vi "Core_2018-02-21.vi"(5 "Error In":errorcluster) -> (19 "Error Out":errorcluster)   [LabVIEW 2017]
uses:
  <vilib>/Platform/TimedLoop/XDataNode/timing_clust.ctl
  <vilib>/Platform/TimedLoop/XDataNode/nitl_modes.ctl
  <vilib>/Platform/TimedLoop/XDataNode/wakeup.ctl
  <vilib>/Platform/TimedLoop/XDataNode/XDataNode.xnode
  <vilib>/Platform/TimedLoop/XDataNode/XDNodeRunTimeDep.lvlib
panel:
  out "Heater Resistance":dbl
  # "Core Module DIagnostics"
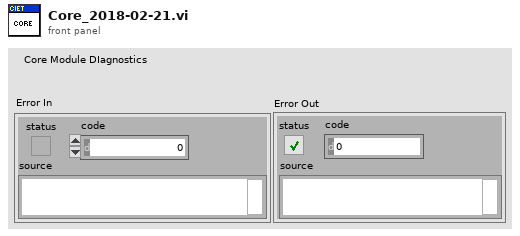
[diagram p1: front panel]
types:
  T1 = typedef "XDNodeRunTimeDep.lvlib/timing_clust.ctl" = cluster{"Expected End [f-1]":u64, "Actual End [f-1]":u64, "Finished Late? [f-1]":bool, "Expected End [i-1]":u64, "Actual End [i-1]":u64, "Finished Late? [i-1]":bool, "Expected Start [i]":u64, "Actual Start [i]":u64, "Expected Start [f]":u64, "Actual Start [f]":u64, "Source Name":string, "Structure Name":string, "Period":i64, "Deadline":i64, "Offset":i64, "Start":i64, "Priority":i32, "Timeout":i32, "Mode":T2, "Wakeup Reason":T3, "Error":errorcluster, "Source Type":string, "Secondary Source Type":string, "Global End Time":u64, "Global Start Time":u64, "Frame Duration":u64, "Iteration Duration":u64, "Assigned CPU":i32, "I/O Scan Engine Mode":u32}
  T2 = typedef "XDNodeRunTimeDep.lvlib/nitl_modes.ctl" = enum32{"No Change", "Process missed periods, maintain original phase", "Discard missed periods, maintain original phase", "Process missed periods, ignore original phase", "Discard missed periods, ignore original phase"}
  T3 = typedef "XDNodeRunTimeDep.lvlib/wakeup.ctl" = enum32{"Normal", "Aborted", "Asynchronous wakeup", "Timing source error", "Timed loop error", "Timeout"}
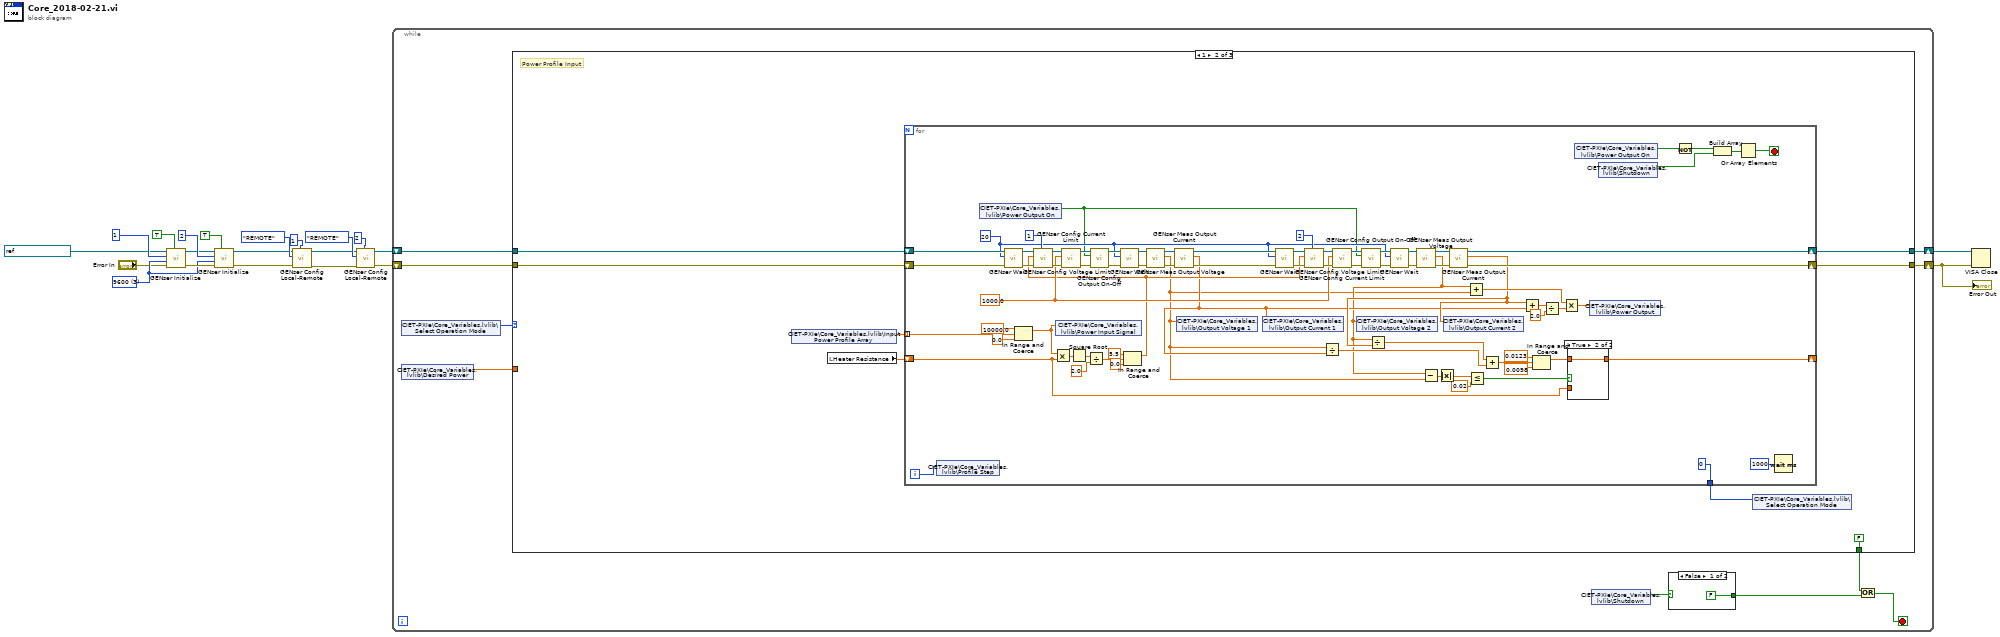
[diagram p0: block diagram]
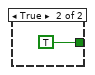
[diagram p2: hidden frame]
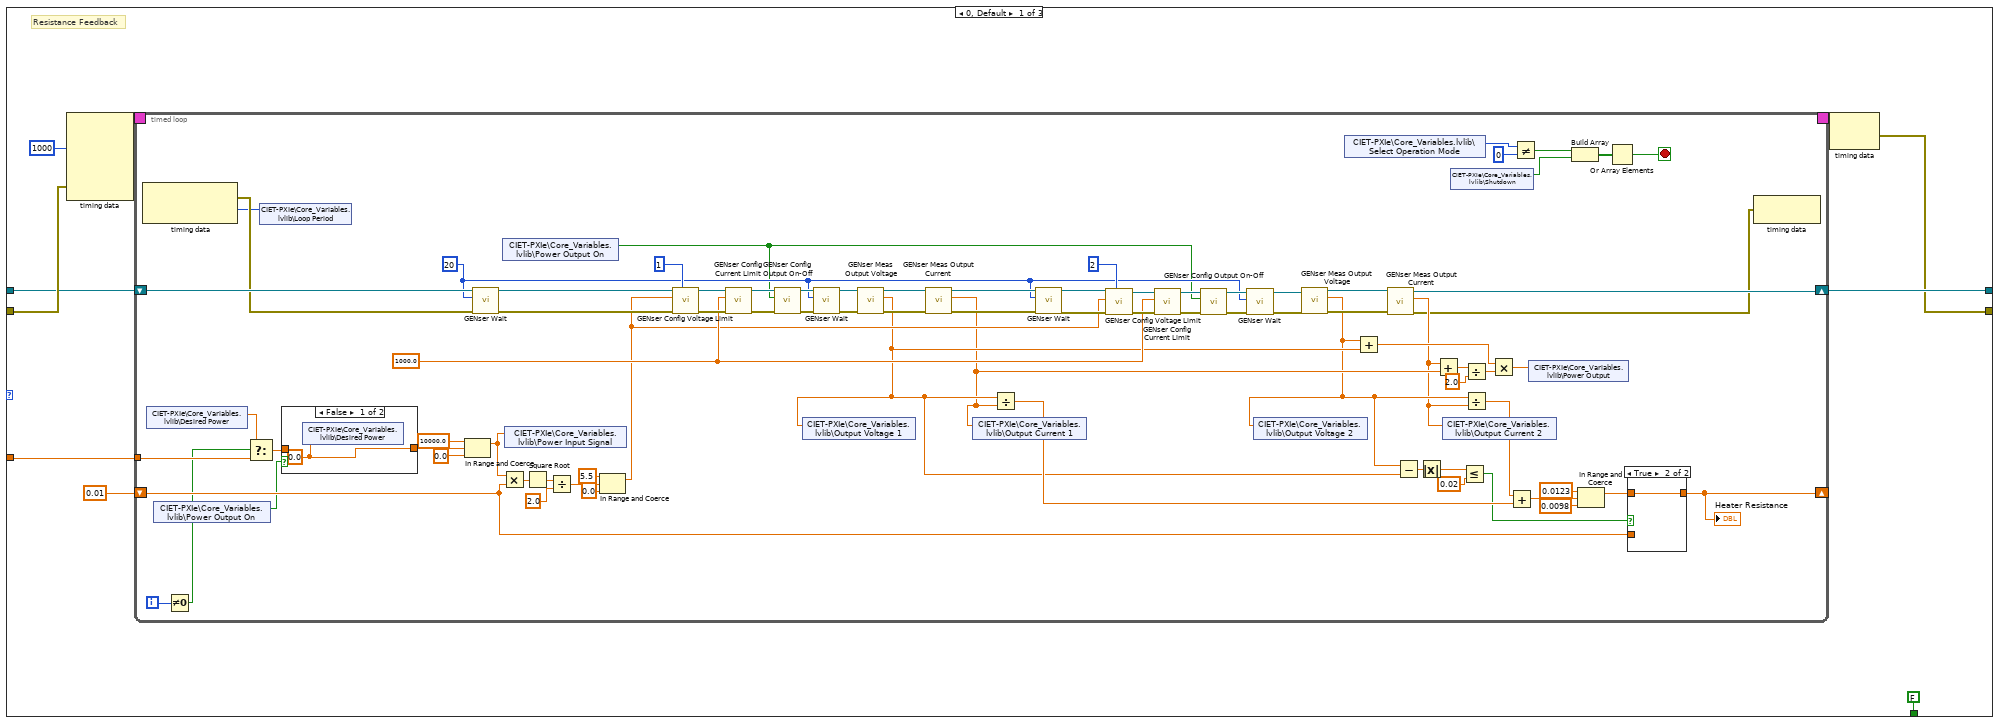
[diagram p3: hidden frame]
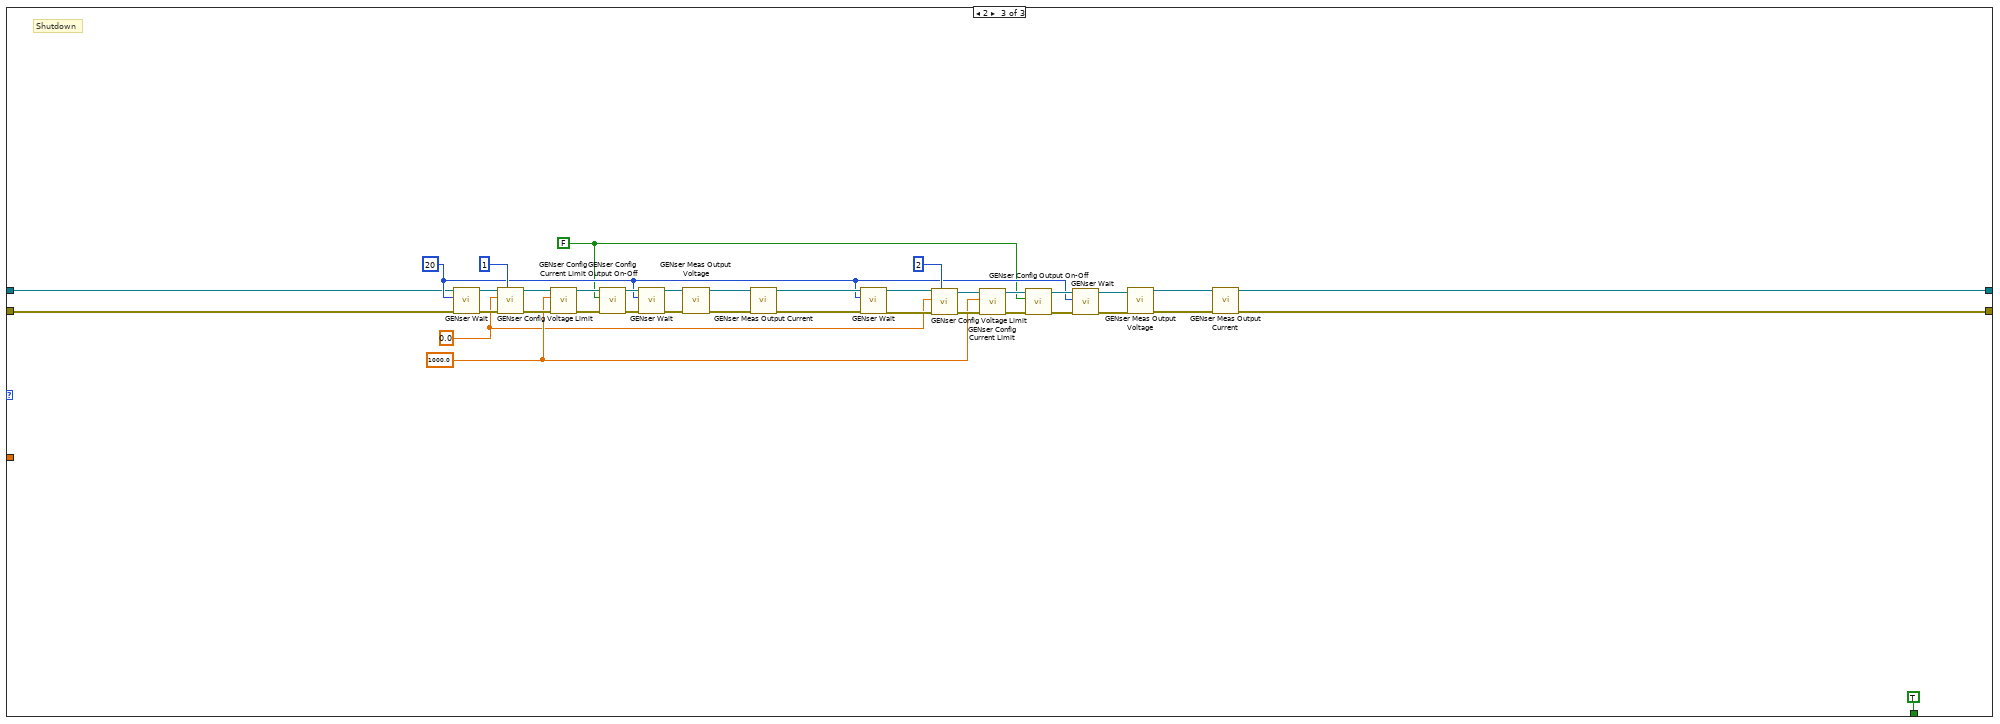
[diagram p7: hidden frame]
diagram:
  w7 = u16 3 items=["1200", "2400", "4800", "9600", "19200"] ("BAUD")
  n1 = call "GENser Initialize.vi"("Reset (T)"=TRUE, "error in (no error)"="Error In", "BAUD"=w7, "GEN Addr"=i16 1, "VISA name"=refnum<visa-resource-name> "Power_Supplies") -> ("error out"=w16:errorcluster, "VISA out"=w17:refnum<visa-resource-name>)  [unwired: 5 in]
  n2 = call "GENser Initialize.vi"("Reset (T)"=TRUE, "error in (no error)"=w16, "BAUD"=w7, "GEN Addr"=i16 2, "VISA name"=w17) -> ("error out"=w13:errorcluster, "VISA out"=w14:refnum<visa-resource-name>)  [unwired: 5 in]
  n3 = call "GENser Config Local-Remote.vi"("GEN Addr"=i16 1, "error"=w13, "Mode"=enum16{"LOCAL", "REMOTE", "LOCKOUT"}."REMOTE", "VISA"=w14) -> ("error out"=w8:errorcluster, "VISA out"=w9:refnum<visa-resource-name>)  [unwired: 6 in]
  n4 = call "GENser Config Local-Remote.vi"("GEN Addr"=i16 2, "error"=w8, "Mode"=enum16{"LOCAL", "REMOTE", "LOCKOUT"}."REMOTE", "VISA"=w9) -> ("error out"=w5:errorcluster, "VISA out"=w4:refnum<visa-resource-name>)  [unwired: 6 in]
  n5 = while {
    shift-right: [w28] -> w1
    shift-left: w5 -> [w31]
    shift-right: [w29] -> w2
    shift-left: w4 -> [w30]
    stop <- w22 stop-if-true
    n6 = shared-variable "CIET-PXIe\\Core_Variables.lvlib\\Select Operation Mode"() -> (w27:i32)  [unwired: 1 in, 1 out]
    n7 = shared-variable "CIET-PXIe\\Core_Variables.lvlib\\Desired Power"() -> (w26:dbl)  [unwired: 1 in, 1 out]
    n8 = case shown="1" w27 {
      tunnel: w31 -> [w41 w144 w228]
      tunnel: w30 -> [w40 w147 w227]
      tunnel: [w38 w146 w226] -> w29
      tunnel: [w37 w143 w225] -> w28
      tunnel: [FALSE ("Shutdown") FALSE ("Shutdown") TRUE ("Shutdown")] -> w24
      tunnel: w26 -> [w35 _ _]
      frame 0, Default {
        # "Resistance Feedback"
        n9 = node-c288(i64 1000 ("Period"), w41) -> (w43:T1)  [unwired: 3 in]
        n10 = timed-loop {
          timing: w43 -> [_]
          timing-out: [_] -> w42
          shift-right: [w45] -> w38
          shift-left: w40 -> [w110]
          shift-right: [w66] -> _
          shift-left: 0.01 -> [w77]
          tunnel: w35 -> [w62]
          i -> [w64]
          stop <- w58 stop-if-true
          w82 = u32 20 ("Delay (20 mS)")
          w95 = 1000.0 ("Current Limit")
          n11 = node-c288() -> (w109:errorcluster, w56:i64)  [unwired: 1 in]
          n12 = shared-variable "CIET-PXIe\\Core_Variables.lvlib\\Desired Power"() -> (w57:dbl)  [unwired: 1 in, 1 out]
          n13 = shared-variable "CIET-PXIe\\Core_Variables.lvlib\\Power Output On"() -> (w54:bool)  [unwired: 1 in, 1 out]
          n14 = Not Equal To 0?(x=w64) -> (x != 0?=w61:bool)
          n15 = Select(t=w57, s=w61, f=w62) -> (s? t:f=w63:dbl)
          n16 = shared-variable "CIET-PXIe\\Core_Variables.lvlib\\Loop Period"(w56) -> ()  [unwired: 1 in, 1 out]
          n17 = case shown="False" w54 {
            tunnel: [w124 w125] -> w86
            tunnel: w63 -> [_ w125]
            frame False {
              w124 = 0.0 ("Desired Power")
              n18 = shared-variable "CIET-PXIe\\Core_Variables.lvlib\\Desired Power"(w124) -> ()  [unwired: 1 in, 1 out]
            }
            frame True {
            }
          }
          n19 = In Range and Coerce(upper limit=10000.0, x=w86, lower limit=0.0) -> (coerced(x)=w53:dbl)  [unwired: 1 out]
          n20 = call "GENser Wait.vi"("error"=w109, "Delay (20 mS)"=w82, "VISA"=w110) -> ("error out"=w111:errorcluster, "VISA out"=w108:refnum<visa-resource-name>)  [unwired: 7 in]
          n21 = Multiply(x=w53, y=w77) -> (x*y=w92:dbl)
          n22 = shared-variable "CIET-PXIe\\Core_Variables.lvlib\\Power Output On"() -> (w55:bool)  [unwired: 1 in, 1 out]
          n23 = shared-variable "CIET-PXIe\\Core_Variables.lvlib\\Power Input Signal"(w53) -> ()  [unwired: 1 in, 1 out]
          n24 = Square Root(x=w92) -> (sqrt(x)=w91:dbl)
          n25 = Divide(x=w91, y=2.0) -> (x/y=w87:dbl)
          n26 = In Range and Coerce(upper limit=5.5, x=w87, lower limit=0.0) -> (coerced(x)=w85:dbl)  [unwired: 1 out]
          n27 = call "GENser Config Voltage Limit.vi"("GEN Addr"=i16 1, "error"=w111, "Volt Limit"=w85, "VISA"=w108) -> ("error out"=w123:errorcluster, "VISA out"=w107:refnum<visa-resource-name>)  [unwired: 6 in]
          n28 = call "GENser Config Current Limit.vi"("error"=w123, "Current Limit"=w95, "VISA"=w107) -> ("error out"=w120:errorcluster, "VISA out"=w106:refnum<visa-resource-name>)  [unwired: 7 in]
          n29 = call "GENser Config Output On-Off.vi"("error"=w120, "Output ON"=w55, "VISA"=w106) -> ("error out"=w118:errorcluster, "VISA out"=w105:refnum<visa-resource-name>)  [unwired: 7 in]
          n30 = call "GENser Wait.vi"("error"=w118, "Delay (20 mS)"=w82, "VISA"=w105) -> ("error out"=w117:errorcluster, "VISA out"=w104:refnum<visa-resource-name>)  [unwired: 7 in]
          n31 = call "GENser Meas Output Voltage.vi"("error"=w117, "VISA"=w104) -> ("error out"=w119:errorcluster, "Output Voltage"=w50:dbl, "VISA out"=w103:refnum<visa-resource-name>)  [unwired: 7 in]
          n32 = shared-variable "CIET-PXIe\\Core_Variables.lvlib\\Output Voltage 1"(w50) -> ()  [unwired: 1 in, 1 out]
          n33 = call "GENser Meas Output Current.vi"("error"=w119, "VISA"=w103) -> ("error out"=w115:errorcluster, "Output Current"=w49:dbl, "VISA out"=w102:refnum<visa-resource-name>)  [unwired: 7 in]
          n34 = shared-variable "CIET-PXIe\\Core_Variables.lvlib\\Output Current 1"(w49) -> ()  [unwired: 1 in, 1 out]
          n35 = Divide(x=w50, y=w49) -> (x/y=w69:dbl)
          n36 = call "GENser Wait.vi"("error"=w115, "Delay (20 mS)"=w82, "VISA"=w102) -> ("error out"=w114:errorcluster, "VISA out"=w101:refnum<visa-resource-name>)  [unwired: 7 in]
          n37 = call "GENser Config Voltage Limit.vi"("GEN Addr"=i16 2, "error"=w114, "Volt Limit"=w85, "VISA"=w101) -> ("error out"=w116:errorcluster, "VISA out"=w100:refnum<visa-resource-name>)  [unwired: 6 in]
          n38 = call "GENser Config Current Limit.vi"("error"=w116, "Current Limit"=w95, "VISA"=w100) -> ("error out"=w113:errorcluster, "VISA out"=w99:refnum<visa-resource-name>)  [unwired: 7 in]
          n39 = call "GENser Config Output On-Off.vi"("error"=w113, "Output ON"=w55, "VISA"=w99) -> ("error out"=w122:errorcluster, "VISA out"=w98:refnum<visa-resource-name>)  [unwired: 7 in]
          n40 = call "GENser Wait.vi"("error"=w122, "Delay (20 mS)"=w82, "VISA"=w98) -> ("error out"=w112:errorcluster, "VISA out"=w97:refnum<visa-resource-name>)  [unwired: 7 in]
          n41 = call "GENser Meas Output Voltage.vi"("error"=w112, "VISA"=w97) -> ("error out"=w121:errorcluster, "Output Voltage"=w48:dbl, "VISA out"=w96:refnum<visa-resource-name>)  [unwired: 7 in]
          n42 = shared-variable "CIET-PXIe\\Core_Variables.lvlib\\Output Voltage 2"(w48) -> ()  [unwired: 1 in, 1 out]
          n43 = shared-variable "CIET-PXIe\\Core_Variables.lvlib\\Select Operation Mode"() -> (w52:i32)  [unwired: 1 in, 1 out]
          n44 = Add(x=w48, y=w50) -> (x+y=w78:dbl)
          n45 = call "GENser Meas Output Current.vi"("error"=w121, "VISA"=w96) -> ("error out"=w44:errorcluster, "Output Current"=w47:dbl, "VISA out"=w45:refnum<visa-resource-name>)  [unwired: 7 in]
          n46 = Subtract(x=w48, y=w50) -> (x-y=w73:dbl)
          n47 = Absolute Value(x=w73) -> (abs(x)=w72:dbl)
          n48 = Add(x=w47, y=w49) -> (x+y=w81:dbl)
          n49 = shared-variable "CIET-PXIe\\Core_Variables.lvlib\\Output Current 2"(w47) -> ()  [unwired: 1 in, 1 out]
          n50 = shared-variable "CIET-PXIe\\Core_Variables.lvlib\\Shutdown"() -> (w51:bool)  [unwired: 1 in, 1 out]
          n51 = Less Or Equal?(x=w72, y=0.02) -> (x <= y?=w68:bool)
          n52 = Divide(x=w81, y=2.0) -> (x/y=w79:dbl)
          n53 = Divide(x=w48, y=w47) -> (x/y=w70:dbl)
          n54 = Multiply(x=w78, y=w79) -> (x*y=w46:dbl)
          n55 = Add(x=w70, y=w69) -> (x+y=w74:dbl)
          n56 = Not Equal?(x=w52, y=u16 0) -> (x != y?=w60:bool)
          n57 = shared-variable "CIET-PXIe\\Core_Variables.lvlib\\Power Output"(w46) -> ()  [unwired: 1 in, 1 out]
          n58 = Build Array(w60, w51) -> (w59:bool[])
          n59 = In Range and Coerce(upper limit=0.0123, x=w74, lower limit=0.0098) -> (coerced(x)=w67:dbl)  [unwired: 1 out]
          n60 = Or Array Elements(Boolean array=w59) -> (logical OR=w58:bool)
          n61 = case shown="True" w68 {
            tunnel: w67 -> [_ w133]
            tunnel: [w132 w133] -> w66
            tunnel: w77 -> [w132 _]
            frame False {
            }
            frame True {
            }
          }
          "Heater Resistance" <- w66
          n62 = node-c288(w44) -> ()  [unwired: 1 out]
        }
        n63 = node-c288(w42) -> (w37:errorcluster)
      }
      frame 1 {
        # "Power Profile Input"
        n64 = shared-variable "CIET-PXIe\\Core_Variables.lvlib\\Input Power Profile Array"() -> (w140:dbl[])  [unwired: 1 in, 1 out]
        n65 = local read "Heater Resistance"() -> (w145:dbl)
        n66 = for {
          shift-right: [w169] -> w146
          shift-left: w147 -> [w209]
          shift-right: [w168] -> w143
          shift-left: w144 -> [w177]
          tunnel: w140 -> [w174] mode=indexing
          tunnel: [u16 0 ("y")] -> w141
          shift-right: [w149] -> _
          shift-left: w145 -> [w148]
          i -> [w164]
          stop <- w175 stop-if-true
          w184 = u32 20 ("Delay (20 mS)")
          w195 = 1000.0 ("Current Limit")
          n67 = shared-variable "CIET-PXIe\\Core_Variables.lvlib\\Profile Step"(w164) -> ()  [unwired: 1 in, 1 out]
          n68 = shared-variable "CIET-PXIe\\Core_Variables.lvlib\\Power Output On"() -> (w171:bool)  [unwired: 1 in, 1 out]
          n69 = call "GENser Wait.vi"("error"=w177, "Delay (20 mS)"=w184, "VISA"=w209) -> ("error out"=w210:errorcluster, "VISA out"=w208:refnum<visa-resource-name>)  [unwired: 7 in]
          n70 = In Range and Coerce(upper limit=10000.0, x=w174, lower limit=0.0) -> (coerced(x)=w172:dbl)  [unwired: 1 out]
          n71 = Multiply(x=w172, y=w148) -> (x*y=w192:dbl)
          n72 = shared-variable "CIET-PXIe\\Core_Variables.lvlib\\Power Input Signal"(w172) -> ()  [unwired: 1 in, 1 out]
          n73 = Square Root(x=w192) -> (sqrt(x)=w191:dbl)
          n74 = Divide(x=w191, y=2.0) -> (x/y=w187:dbl)
          n75 = In Range and Coerce(upper limit=5.5, x=w187, lower limit=0.0) -> (coerced(x)=w179:dbl)  [unwired: 1 out]
          n76 = call "GENser Config Voltage Limit.vi"("GEN Addr"=i16 1, "error"=w210, "Volt Limit"=w179, "VISA"=w208) -> ("error out"=w222:errorcluster, "VISA out"=w207:refnum<visa-resource-name>)  [unwired: 6 in]
          n77 = call "GENser Config Current Limit.vi"("error"=w222, "Current Limit"=w195, "VISA"=w207) -> ("error out"=w219:errorcluster, "VISA out"=w206:refnum<visa-resource-name>)  [unwired: 7 in]
          n78 = call "GENser Config Output On-Off.vi"("error"=w219, "Output ON"=w171, "VISA"=w206) -> ("error out"=w217:errorcluster, "VISA out"=w205:refnum<visa-resource-name>)  [unwired: 7 in]
          n79 = call "GENser Wait.vi"("error"=w217, "Delay (20 mS)"=w184, "VISA"=w205) -> ("error out"=w216:errorcluster, "VISA out"=w204:refnum<visa-resource-name>)  [unwired: 7 in]
          n80 = call "GENser Meas Output Voltage.vi"("error"=w216, "VISA"=w204) -> ("error out"=w218:errorcluster, "Output Voltage"=w150:dbl, "VISA out"=w203:refnum<visa-resource-name>)  [unwired: 7 in]
          n81 = call "GENser Meas Output Current.vi"("error"=w218, "VISA"=w203) -> ("error out"=w214:errorcluster, "Output Current"=w154:dbl, "VISA out"=w202:refnum<visa-resource-name>)  [unwired: 7 in]
          n82 = shared-variable "CIET-PXIe\\Core_Variables.lvlib\\Output Voltage 1"(w150) -> ()  [unwired: 1 in, 1 out]
          n83 = shared-variable "CIET-PXIe\\Core_Variables.lvlib\\Output Current 1"(w154) -> ()  [unwired: 1 in, 1 out]
          n84 = call "GENser Wait.vi"("error"=w214, "Delay (20 mS)"=w184, "VISA"=w202) -> ("error out"=w213:errorcluster, "VISA out"=w201:refnum<visa-resource-name>)  [unwired: 7 in]
          n85 = call "GENser Config Voltage Limit.vi"("GEN Addr"=i16 2, "error"=w213, "Volt Limit"=w179, "VISA"=w201) -> ("error out"=w215:errorcluster, "VISA out"=w200:refnum<visa-resource-name>)  [unwired: 6 in]
          n86 = Divide(x=w150, y=w154) -> (x/y=w152:dbl)
          n87 = call "GENser Config Current Limit.vi"("error"=w215, "Current Limit"=w195, "VISA"=w200) -> ("error out"=w212:errorcluster, "VISA out"=w199:refnum<visa-resource-name>)  [unwired: 7 in]
          n88 = call "GENser Config Output On-Off.vi"("error"=w212, "Output ON"=w171, "VISA"=w199) -> ("error out"=w221:errorcluster, "VISA out"=w198:refnum<visa-resource-name>)  [unwired: 7 in]
          n89 = call "GENser Wait.vi"("error"=w221, "Delay (20 mS)"=w184, "VISA"=w198) -> ("error out"=w211:errorcluster, "VISA out"=w197:refnum<visa-resource-name>)  [unwired: 7 in]
          n90 = call "GENser Meas Output Voltage.vi"("error"=w211, "VISA"=w197) -> ("error out"=w220:errorcluster, "Output Voltage"=w151:dbl, "VISA out"=w196:refnum<visa-resource-name>)  [unwired: 7 in]
          n91 = shared-variable "CIET-PXIe\\Core_Variables.lvlib\\Output Voltage 2"(w151) -> ()  [unwired: 1 in, 1 out]
          n92 = Subtract(x=w151, y=w150) -> (x-y=w160:dbl)
          n93 = Absolute Value(x=w160) -> (abs(x)=w159:dbl)
          n94 = call "GENser Meas Output Current.vi"("error"=w220, "VISA"=w196) -> ("error out"=w168:errorcluster, "Output Current"=w155:dbl, "VISA out"=w169:refnum<visa-resource-name>)  [unwired: 7 in]
          n95 = Divide(x=w151, y=w155) -> (x/y=w153:dbl)
          n96 = shared-variable "CIET-PXIe\\Core_Variables.lvlib\\Output Current 2"(w155) -> ()  [unwired: 1 in, 1 out]
          n97 = Add(x=w151, y=w150) -> (x+y=w180:dbl)
          n98 = Less Or Equal?(x=w159, y=0.02) -> (x <= y?=w157:bool)
          n99 = Add(x=w153, y=w152) -> (x+y=w161:dbl)
          n100 = Add(x=w155, y=w154) -> (x+y=w183:dbl)
          n101 = In Range and Coerce(upper limit=0.0123, x=w161, lower limit=0.0098) -> (coerced(x)=w156:dbl)  [unwired: 1 out]
          n102 = Divide(x=w183, y=2.0) -> (x/y=w181:dbl)
          n103 = Multiply(x=w180, y=w181) -> (x*y=w170:dbl)
          n104 = case shown="True" w157 {
            tunnel: w156 -> [_ w224]
            tunnel: [w223 w224] -> w149
            tunnel: w148 -> [w223 _]
            frame False {
            }
            frame True {
            }
          }
          n105 = shared-variable "CIET-PXIe\\Core_Variables.lvlib\\Power Output On"() -> (w167:bool)  [unwired: 1 in, 1 out]
          n106 = shared-variable "CIET-PXIe\\Core_Variables.lvlib\\Power Output"(w170) -> ()  [unwired: 1 in, 1 out]
          n107 = shared-variable "CIET-PXIe\\Core_Variables.lvlib\\Shutdown"() -> (w166:bool)  [unwired: 1 in, 1 out]
          n108 = Not(x=w167) -> (.not. x?=w173:bool)
          n109 = Build Array(w173, w166) -> (w178:bool[])
          n110 = Or Array Elements(Boolean array=w178) -> (logical OR=w175:bool)
          n111 = Wait (ms)(milliseconds to wait=u32 1000) -> ()  [unwired: 1 out]
        }
        n112 = shared-variable "CIET-PXIe\\Core_Variables.lvlib\\Select Operation Mode"(w141) -> ()  [unwired: 1 in, 1 out]
      }
      frame 2 {
        w229 = 0.0 ("Volt Limit")
        w231 = FALSE ("Output ON")
        w232 = u32 20 ("Delay (20 mS)")
        w230 = 1000.0 ("Current Limit")
        # "Shutdown"
        n113 = call "GENser Wait.vi"("error"=w228, "Delay (20 mS)"=w232, "VISA"=w227) -> ("error out"=w248:errorcluster, "VISA out"=w247:refnum<visa-resource-name>)  [unwired: 7 in]
        n114 = call "GENser Config Voltage Limit.vi"("GEN Addr"=i16 1, "error"=w248, "Volt Limit"=w229, "VISA"=w247) -> ("error out"=w260:errorcluster, "VISA out"=w246:refnum<visa-resource-name>)  [unwired: 6 in]
        n115 = call "GENser Config Current Limit.vi"("error"=w260, "Current Limit"=w230, "VISA"=w246) -> ("error out"=w257:errorcluster, "VISA out"=w245:refnum<visa-resource-name>)  [unwired: 7 in]
        n116 = call "GENser Config Output On-Off.vi"("error"=w257, "Output ON"=w231, "VISA"=w245) -> ("error out"=w255:errorcluster, "VISA out"=w244:refnum<visa-resource-name>)  [unwired: 7 in]
        n117 = call "GENser Wait.vi"("error"=w255, "Delay (20 mS)"=w232, "VISA"=w244) -> ("error out"=w254:errorcluster, "VISA out"=w243:refnum<visa-resource-name>)  [unwired: 7 in]
        n118 = call "GENser Meas Output Voltage.vi"("error"=w254, "VISA"=w243) -> ("error out"=w256:errorcluster, "VISA out"=w242:refnum<visa-resource-name>)  [unwired: 7 in, 1 out]
        n119 = call "GENser Meas Output Current.vi"("error"=w256, "VISA"=w242) -> ("error out"=w252:errorcluster, "VISA out"=w241:refnum<visa-resource-name>)  [unwired: 7 in, 1 out]
        n120 = call "GENser Wait.vi"("error"=w252, "Delay (20 mS)"=w232, "VISA"=w241) -> ("error out"=w251:errorcluster, "VISA out"=w240:refnum<visa-resource-name>)  [unwired: 7 in]
        n121 = call "GENser Config Voltage Limit.vi"("GEN Addr"=i16 2, "error"=w251, "Volt Limit"=w229, "VISA"=w240) -> ("error out"=w253:errorcluster, "VISA out"=w239:refnum<visa-resource-name>)  [unwired: 6 in]
        n122 = call "GENser Config Current Limit.vi"("error"=w253, "Current Limit"=w230, "VISA"=w239) -> ("error out"=w250:errorcluster, "VISA out"=w238:refnum<visa-resource-name>)  [unwired: 7 in]
        n123 = call "GENser Config Output On-Off.vi"("error"=w250, "Output ON"=w231, "VISA"=w238) -> ("error out"=w259:errorcluster, "VISA out"=w237:refnum<visa-resource-name>)  [unwired: 7 in]
        n124 = call "GENser Wait.vi"("error"=w259, "Delay (20 mS)"=w232, "VISA"=w237) -> ("error out"=w249:errorcluster, "VISA out"=w236:refnum<visa-resource-name>)  [unwired: 7 in]
        n125 = call "GENser Meas Output Voltage.vi"("error"=w249, "VISA"=w236) -> ("error out"=w258:errorcluster, "VISA out"=w235:refnum<visa-resource-name>)  [unwired: 7 in, 1 out]
        n126 = call "GENser Meas Output Current.vi"("error"=w258, "VISA"=w235) -> ("error out"=w225:errorcluster, "VISA out"=w226:refnum<visa-resource-name>)  [unwired: 7 in, 1 out]
      }
    }
    n127 = shared-variable "CIET-PXIe\\Core_Variables.lvlib\\Shutdown"() -> (w25:bool)  [unwired: 1 in, 1 out]
    n128 = case shown="False" w25 {
      tunnel: [FALSE ("Shutdown") TRUE ("Shutdown")] -> w23
      frame False {
      }
      frame True {
      }
    }
    n129 = Or(x=w24, y=w23) -> (x .or. y?=w22:bool)
  }
  "Error Out" <- w1
  n130 = VISA Close(VISA resource name=w2, error in (no error)=w1) -> ()  [unwired: 1 out]
